vi "direct_ads_sur_piStar_pyxgTpsatM.vi"(0 "WorkingPair (Input)":T1={"no_iso"=1, "no_p_sat"=1, "path_db"="D:\\Driesel\\SorpLibLocal\\LabVIEW_wrapper\\data\\json\\sorpproplib_minimalExample.json", "wp_as"="silicagel", "wp_st"="123", "wp_iso"="DubininArctan1", "wp_rf"="water", "rf_rhol"="SaturatedLiquidDensity_EoS1", "no_rhol"=1, "rf_psat"="VaporPressure_EoS1"}, 1 "Molar fraction of refrigerant in adsorbed phase in mol/mol (Input)":dbl, 2 "Molar fraction of refrigerant in vapor phase in mol/mol (Input)":dbl, 3 "Total pressure of vapor phase in Pa (Input)":dbl, 5 "Temperature in K (Input)":dbl, 7 "Activity coefficient of refrigerant in adsorbed phase (Input)":dbl, 9 "Saturation vapor pressure in Pa (Input)":dbl, 11 "Error (Input)":errorcluster, 12 "Molar mass of refrigerant M in kg/mol (Input)":dbl) -> (4 "Reduced spreading pressure in kg/mol (Output)":dbl, 15 "Error (Output)":errorcluster caption="Error(Output)")   [LabVIEW 2017]
doc: "direct_ads_sur_piStar_pyxgTpsatM:\n * ---------------------------------\n *\n * Calculates reduced spreading pressure piStar in kg/mol depending on\n * equilibrium pressure p in Pa, molar fraction of refrigerant in vapor phase\n * in mol/mol, molar fraction of refrigerant in adsorbed phase in mol/mol,\n * activity coefficient of refrigerant in adsorbed phase, equilibrium\n * temperature T in K, saturation pressure p_sat in Pa, and molar mass of\n * refrigerant M in kg/mol. The reduced spreading pressure is defined as\n * follows:\n *\n * piStar = A * pi / (R * T * m_sorbent) = 1 / M *\n * Integral_0^p0{w(p,T) / p * dp}\n *\n * where p0 = p_total*y / (gamma*x)\n *\n * Parameters:\n * -----------\n * double p_total_Pa:\n * Total pressure of vapor phase in Pa.\n * double y_molmol:\n * Molar fraction of refrigerant in vapor phase in mol/mol.\n * double x_molmol:\n * Molar fraction of refrigerant in adsorbed phase in mol/mol.\n * double gamma:\n * Activity coefficient of refrigerant in adsorbed phase.\n * double T_K:\n * Equilibrium temperature in K.\n * double p_sat_Pa:\n * Saturation vapor pressure in Pa.\n * double M_kgmol:\n * Molar mass of refrigerant M in kg/mol.\n *\n * const char *path_db:\n * Path to database.\n * const char *wp_as:\n * Name of sorbent.\n * const char *wp_st:\n * Name of sub-type of sorbent.\n * const char *wp_rf:\n * Name of refrigerant.\n * const char *wp_iso:\n * Name of isotherm.\n * int no_iso:\n * ID of isotherm (i.e. when more than one isotherm is available)\n * const char *rf_psat:\n * Name of calculation approach for vapor pressure.\n * int no_p_sat:\n * ID of vapor pressure equation (i.e. when more than one equation is\n * available)\n * const char *rf_rhol:\n * Name of calculation approach for liquid density.\n * int no_rhol:\n * ID of liquid density equation (i.e. when more than one equation is\n * available)\n *\n * Returns:\n * --------\n * double:\n * Reduced spreading pressure in kg/mol.\n *\n * Remarks:\n * --------\n * This function is only valid for isotherm models based on the surface\n * approach using the saturated vapor pressure as additional argument.\n *\n * History:\n * --------\n * 07/07/2021, by Jannik Driesel (supervised by Mirko Engelpracht):\n * First implementation."
uses:
  data/win32bit/libsorpPropLib.dll
panel:
  # "Path to database"
  # "Name of sorbent"
  # "Name of sub-type of sorbent"
  # "Name of refrigerant"
  # "Name of isotherm"
  # "ID of isotherm"
  # "Name of calculation approach for vapor pressure"
  # "ID of vapor pressure equation"
  # "Name of calculation approach for liquid density"
  # "ID of liquid density equation"
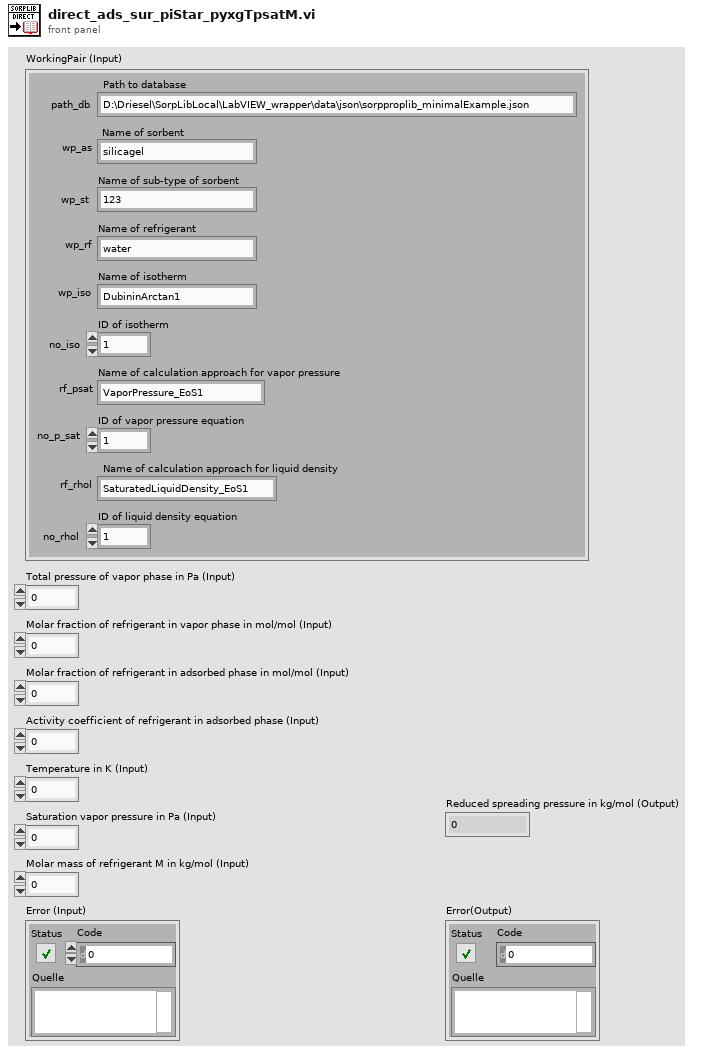
[diagram p1: front panel]
types:
  T1 = cluster{"no_iso":i32, "no_p_sat":i32, "path_db":string, "wp_as":string, "wp_st":string, "wp_iso":string, "wp_rf":string, "rf_rhol":string, "no_rhol":i32, "rf_psat":string}
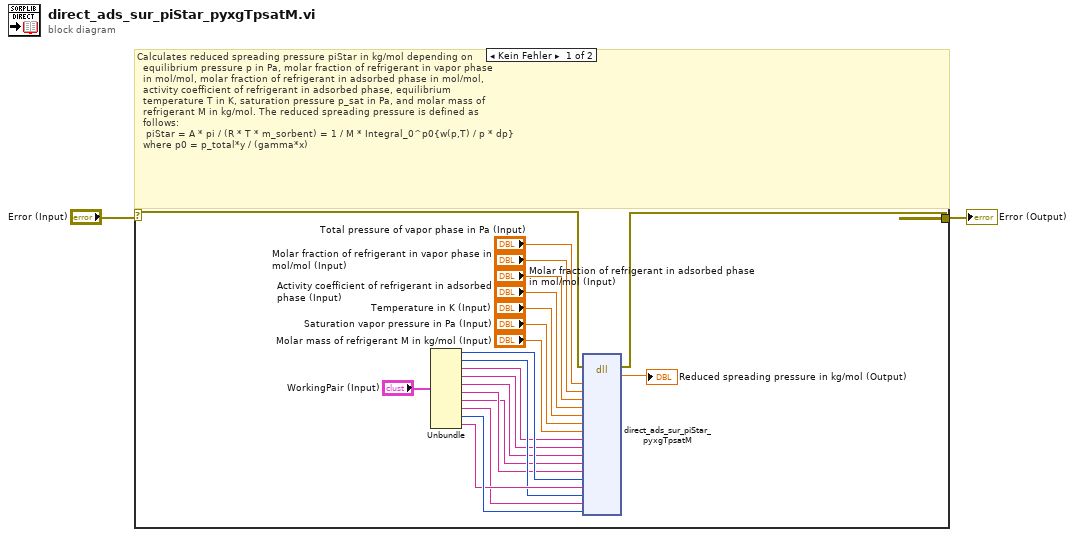
[diagram p0: block diagram]
diagram:
  n1 = case shown="Kein Fehler" "Error (Input)" {
    selector: "Error (Input)" -> [w11 w24]
    tunnel: [w10 w24] -> w1
    frame No Error {
      # "Calculates reduced spreading pressure piStar in kg/mol depending on\n  equilibrium pressure p in Pa, molar fraction of refrigerant in vapor phase\n  in mol/mol, molar fraction of refrigerant in adsorbed phase in mol/mol,\n  activity coefficient of refrigerant in adsorbed phase, equilibrium\n  temperature T in K, saturation pressure p_sat in Pa, and molar mass of\n  refrigerant M in kg/mol. The reduced spreading pressure is defined as\n  follows:\n  \tpiStar = A * pi / (R * T * m_sorbent) = 1 / M *\tIntegral_0^p0{w(p,T) / p * dp}\n \twhere p0 = p_total*y / (gamma*x)"
      n2 = Unbundle("WorkingPair (Input)") -> ("no_iso"=w19:i32, "no_p_sat"=w20:i32, "path_db"=w13:string, "wp_as"=w14:string, "wp_st"=w15:string, "wp_iso"=w17:string, "wp_rf"=w16:string, "rf_rhol"=w18:string, "no_rhol"=w22:i32, "rf_psat"=w21:string)
      n3 = dll-call lib="D:/Driesel/SorpLibLocal/LabVIEW_wrapper/data/win32bit/libsorpPropLib.dll" fn="direct_ads_sur_piStar_pyxgTpsatM"(error in=w11, "p_total_Pa"="Total pressure of vapor phase in Pa (Input)", "y_molmol"="Molar fraction of refrigerant in vapor phase in mol/mol (Input)", "x_molmol"="Molar fraction of refrigerant in adsorbed phase in mol/mol (Input)", "gamma"="Activity coefficient of refrigerant in adsorbed phase (Input)", "T_K"="Temperature in K (Input)", "p_sat_Pa"="Saturation vapor pressure in Pa (Input)", "M_kgmol"="Molar mass of refrigerant M in kg/mol (Input)", "path_db"=w13, "wp_as"=w14, "wp_st"=w15, "wp_rf"=w16, "wp_iso"=w17, "no_iso"=w19, "rf_psat"=w21, "no_p_sat"=w20, "rf_rhol"=w18, "no_rhol"=w22) -> (error out=w10:errorcluster, "piStar_kgmol"=→"Reduced spreading pressure in kg/mol (Output)":dbl)  [unwired: 19 in, 1 out]
    }
    frame Error {
      # "Error - No calculations"
    }
  }
  "Error (Output)" <- w1
